vi "LINC String Parser.vi"(10 "index in":i32, 11 "string in":u8[](array[numeric])) -> (0 "comma found":bool, 1 "string found":string, 2 "index out":i32, 3 "string out":u8[](array[numeric]), 4 "end":bool)   [LabVIEW 2018, in "STEPkgDriver_LINC.lvlib"]
uses:
  STEPkgDriver_LINC.lvlib
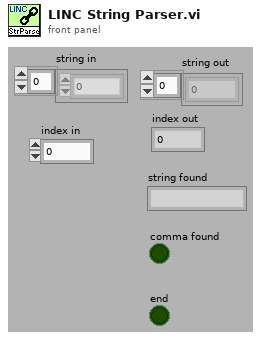
[diagram p1: front panel]
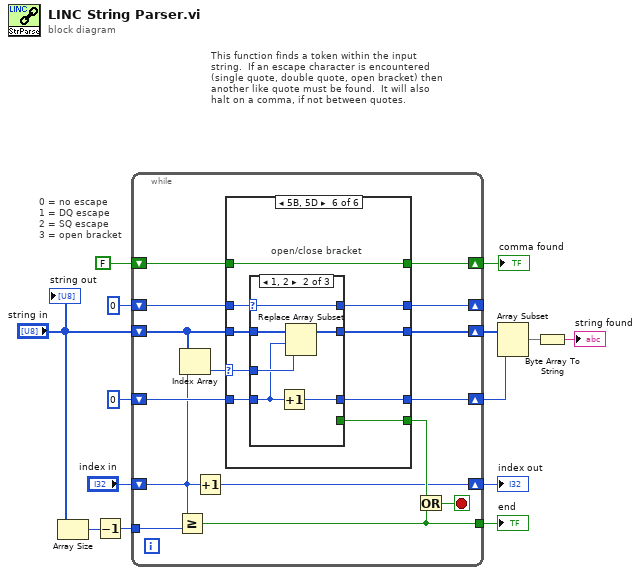
[diagram p0: block diagram]
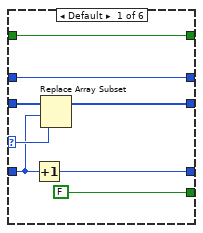
[diagram p2: hidden frame]
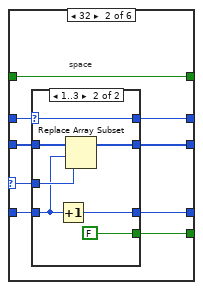
[diagram p3: hidden frame]
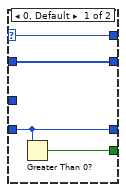
[diagram p4: hidden frame]
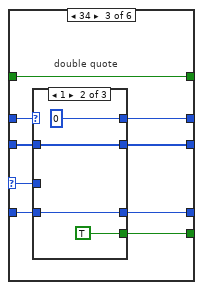
[diagram p5: hidden frame]
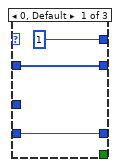
[diagram p6: hidden frame]
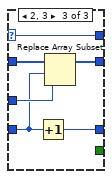
[diagram p7: hidden frame]
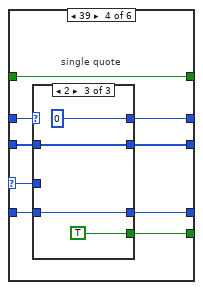
[diagram p8: hidden frame]
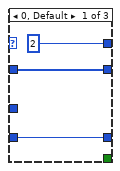
[diagram p9: hidden frame]
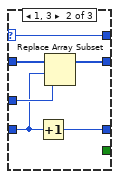
[diagram p10: hidden frame]
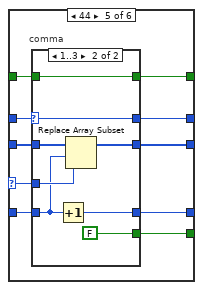
[diagram p11: hidden frame]
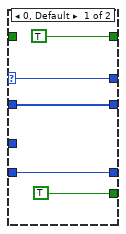
[diagram p12: hidden frame]
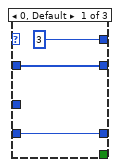
[diagram p13: hidden frame]
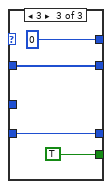
[diagram p14: hidden frame]
diagram:
  # "0 = no escape\n1 = DQ escape\n2 = SQ escape\n3 = open bracket"
  # "This function finds a token within the input string.  If an escape character is encountered (single quote, double quote, open bracket) then another like quote must be found.  It will also halt on a comma, if not between quotes."
  n1 = Array Size(array="string in") -> (size(s)=w13:i32)
  n2 = Decrement(x=w13) -> (x-1=w12:i32)
  n3 = while {
    shift-right: [w27] -> w8
    shift-left: "string in" -> [w28]
    shift-right: [w25] -> _
    shift-left: 0 -> [w26]
    tunnel: w12 -> [w24]
    shift-right: [w21] -> w9
    shift-left: 0 -> [w22]
    shift-right: [w19] -> w4
    shift-left: "index in" -> [w18]
    shift-right: [w16] -> w2
    shift-left: FALSE -> [w17]
    tunnel: [w15] -> w1
    stop <- w23 stop-if-true
    n4 = Greater Or Equal?(x=w18, y=w24) -> (x >= y?=w15:bool)
    n5 = Index Array(array=w28, index=w18) -> (element=w29:u8)
    n6 = Increment(x=w18) -> (x+1=w19:i32)
    n7 = case shown="5B, 5D" w29 {
      selector: w29 -> [w34 w44 w64 w86 w109 w131]
      tunnel: w28 -> [w37 w46 w66 w88 w111 w133]
      tunnel: [w36 w45 w65 w87 w110 w132] -> w27
      tunnel: w26 -> [w35 w41 w61 w83 w106 w128]
      tunnel: [w35 w39 w60 w82 w104 w127] -> w25
      tunnel: [w33 w42 w62 w84 w107 w129] -> w21
      tunnel: w22 -> [w32 w43 w63 w85 w108 w130]
      tunnel: [FALSE w40 w58 w80 w105 w125] -> w20
      tunnel: w17 -> [w30 w38 w59 w81 w103 w126]
      tunnel: [w30 w38 w59 w81 w102 w126] -> w16
      frame Default {
        n8 = Increment(x=w32) -> (x+1=w33:i32)
        n9 = Replace Array Subset(array=w37, new element=w34, index=w32) -> (w36:u8[])
      }
      frame 32 {
        # "space"
        n10 = case shown="1..3" w41 {
          selector: w41 -> [w49 w51]
          tunnel: w46 -> [w50 w57]
          tunnel: [w50 w56] -> w45
          tunnel: w44 -> [_ w55]
          tunnel: w43 -> [w48 w54]
          tunnel: [w48 w53] -> w42
          tunnel: [w47 FALSE] -> w40
          tunnel: [w49 w51] -> w39
          frame 0, Default {
            n11 = Greater Than 0?(x=w48) -> (x > 0?=w47:bool)
          }
          frame 1..3 {
            n12 = Increment(x=w54) -> (x+1=w53:i32)
            n13 = Replace Array Subset(array=w57, new element=w55, index=w54) -> (w56:u8[])
          }
        }
      }
      frame 34 {
        # "double quote"
        n14 = case shown="1" w61 {
          selector: w61 -> [_ _ w74]
          tunnel: w66 -> [w68 w72 w79]
          tunnel: [w68 w72 w78] -> w65
          tunnel: w64 -> [_ _ w77]
          tunnel: w63 -> [w69 w73 w76]
          tunnel: [w69 w73 w75] -> w62
          tunnel: [1 0 w74] -> w60
          tunnel: [_ TRUE _] -> w58
          frame 0, Default {
          }
          frame 1 {
          }
          frame 2, 3 {
            n15 = Increment(x=w76) -> (x+1=w75:i32)
            n16 = Replace Array Subset(array=w79, new element=w77, index=w76) -> (w78:u8[])
          }
        }
      }
      frame 39 {
        # "single quote"
        n17 = case shown="2" w83 {
          selector: w83 -> [_ w92 _]
          tunnel: w88 -> [w90 w97 w100]
          tunnel: [w90 w96 w100] -> w87
          tunnel: w86 -> [_ w95 _]
          tunnel: w85 -> [w91 w94 w101]
          tunnel: [w91 w93 w101] -> w84
          tunnel: [2 w92 0] -> w82
          tunnel: [_ _ TRUE] -> w80
          frame 0, Default {
          }
          frame 1, 3 {
            n18 = Increment(x=w94) -> (x+1=w93:i32)
            n19 = Replace Array Subset(array=w97, new element=w95, index=w94) -> (w96:u8[])
          }
          frame 2 {
          }
        }
      }
      frame 44 {
        # "comma"
        n20 = case shown="1..3" w106 {
          selector: w106 -> [w115 w118]
          tunnel: w111 -> [w116 w124]
          tunnel: [w116 w123] -> w110
          tunnel: w109 -> [_ w122]
          tunnel: w108 -> [w114 w121]
          tunnel: [w114 w120] -> w107
          tunnel: [TRUE FALSE] -> w105
          tunnel: [w115 w118] -> w104
          tunnel: w103 -> [_ w117]
          tunnel: [TRUE w117] -> w102
          frame 0, Default {
          }
          frame 1..3 {
            n21 = Increment(x=w121) -> (x+1=w120:i32)
            n22 = Replace Array Subset(array=w124, new element=w122, index=w121) -> (w123:u8[])
          }
        }
      }
      frame 91, 93 {
        # "open/close bracket"
        n23 = case shown="1, 2" w128 {
          selector: w128 -> [_ w137 _]
          tunnel: w133 -> [w135 w142 w145]
          tunnel: [w135 w141 w145] -> w132
          tunnel: w131 -> [_ w140 _]
          tunnel: w130 -> [w136 w139 w146]
          tunnel: [w136 w138 w146] -> w129
          tunnel: [3 w137 0] -> w127
          tunnel: [_ _ TRUE] -> w125
          frame 0, Default {
          }
          frame 1, 2 {
            n24 = Increment(x=w139) -> (x+1=w138:i32)
            n25 = Replace Array Subset(array=w142, new element=w140, index=w139) -> (w141:u8[])
          }
          frame 3 {
          }
        }
      }
    }
    n26 = Or(x=w20, y=w15) -> (x .or. y?=w23:bool)
  }
  "index out" <- w4
  "comma found" <- w2
  "end" <- w1
  n27 = Array Subset(array=w8, length=w9) -> (w14:u8[])  [unwired: 1 in]
  n28 = Byte Array To String(unsigned byte array=w14) -> (string=→"string found":string)
  "string out" <- "string in"
